vi "ExecuteBuildSpec.vi"(8 "error in (no error)":errorcluster, 10 "Spec Info":T1, 11 "ExecuteAllBuildSpecsWithVersion in":refnum<class "ExecuteAllBuildSpecsWithVersion.lvclass">) -> (0 "error out":errorcluster, 1 "Operation Output/Error Out":string, 2 "CLI Process Return Code":i32, 3 "ExecuteAllBuildSpecsWithVersion out":refnum<class "ExecuteAllBuildSpecsWithVersion.lvclass">)   [LabVIEW 2015, in "ExecuteAllBuildSpecsWithVersion.lvclass"]
doc: "Builds the builds spec in <b>Spec Info</b>."
uses:
  ExecuteAllBuildSpecsWithVersion.lvclass
  ExecuteMultipleBuildSpecs/SpecInformation.ctl
  ExecuteMultipleBuildSpecs/ExecuteMultipleBuildSpecs.lvclass/ExecuteMultipleBuildSpecs.ctl
  <nishared>/LabVIEW CLI/Operations/CoreOperation/CoreOperation.lvclass/CoreOperation.ctl
  ExecuteAllBuildSpecsWithVersion.lvclass/ExecuteAllBuildSpecsWithVersion.ctl
  ExecuteMultipleBuildSpecs/Read Project Path.vi
  <vilib>/AppBuilder/AB_API_Simple/Build (path).vi
  <vilib>/AppBuilder/AB_API_Simple/Set Build Specification Version (path).vi
  <nishared>/LabVIEW CLI/Operations/Utilities/Logger/Logger.lvclass
  <nishared>/LabVIEW CLI/Operations/CoreOperation/CoreOperation.lvclass
  <vilib>/AppBuilder/AB_API_Simple/NI_App_Builder_API.lvlib
  ExecuteMultipleBuildSpecs/ExecuteMultipleBuildSpecs.lvclass
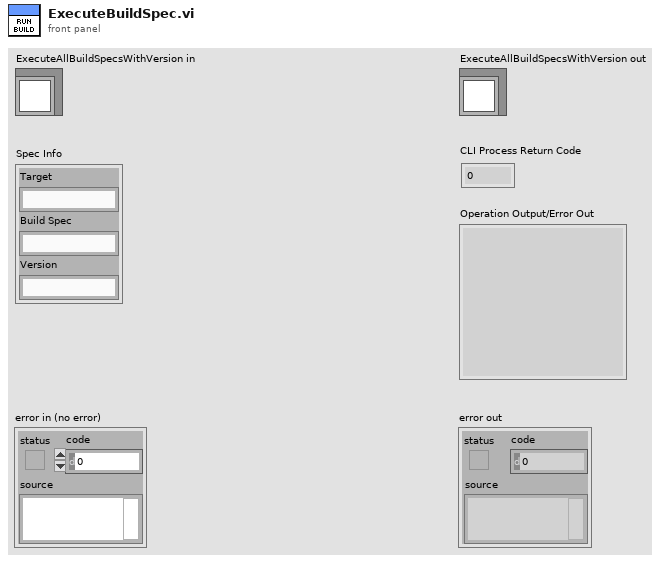
[diagram p1: front panel]
types:
  T1 = typedef "ExecuteMultipleBuildSpecs.lvclass/SpecInformation.ctl" = cluster{"Target":string, "Build Spec":string, "Version":string}
  T2 = typedef "NI_App_Builder_API.lvlib/Build Specification Version.ctl" = cluster{"Major":u16, "Minor":u16, "Fix":u16, "Build":u16}
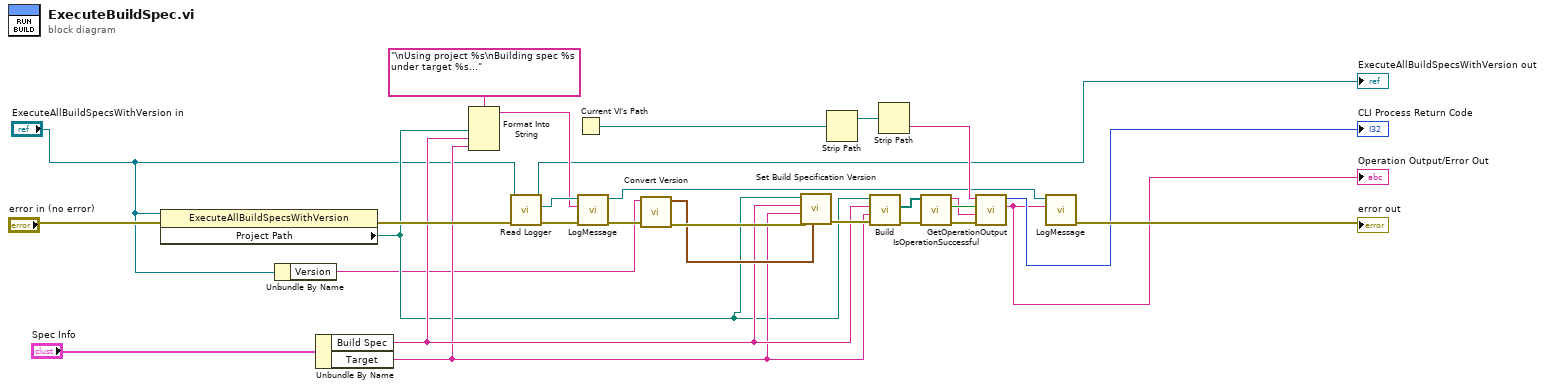
[diagram p0: block diagram]
diagram:
  n1 = property class="ExecuteAllBuildSpecsWithVersion"(reference="ExecuteAllBuildSpecsWithVersion in", error in="error in (no error)") -> (error out=w10:errorcluster, "Project Path"=w3:path)  [unwired: 1 out]
  n2 = Unbundle By Name("ExecuteAllBuildSpecsWithVersion in") -> ("Version"=w1:string)
  n3 = Unbundle By Name("Spec Info") -> ("Build Spec"=w5:string, "Target"=w4:string)
  n4 = Format Into String(format string="\nUsing project %s\nBuilding spec %s under target %s...", w3, w5, w4) -> (resulting string=w26:string)  [unwired: 2 in, 1 out]
  n5 = call <nishared>:"Read Logger.vi"("error in (no error)"=w10, "CoreOperation in"="ExecuteAllBuildSpecsWithVersion in") -> ("error out"=w29:errorcluster, "Logger.lvclass"=w28:refnum<class "Logger.lvclass">, "CoreOperation out"=→"ExecuteAllBuildSpecsWithVersion out":refnum<class "ExecuteAllBuildSpecsWithVersion.lvclass">)  [unwired: 7 in]
  n6 = Current VI's Path() -> (path=w22:path)
  n7 = call <nishared>:"LogMessage.vi"("error in (no error)"=w29, "Message"=w26, "Logger in"=w28) -> ("error out"=w7:errorcluster, "Logger out"=w18:refnum<class "Logger.lvclass">)  [unwired: 7 in]
  n8 = call "Convert Version.vi"("error in (no error)"=w7, "Version"=w1) -> ("error out"=w9:errorcluster, "Build Specification Version"=w8:T2)  [unwired: 8 in]
  n9 = call-poly <vilib>:"Set Build Specification Version.vi"("Build Specification Version"=w8, "error in (no error)"=w9, "Name of target (My Computer)"=w4, "Name of build specification"=w5, "Path to project"=w3) -> ("error out"=w6:errorcluster)  [unwired: 6 in]
  n10 = Strip Path(path=w22) -> (stripped path=w23:path)  [unwired: 1 out]
  n11 = call-poly <vilib>:"Build.vi"("error in (no error)"=w6, "Name of target (My Computer)"=w4, "Name of build specification (if empty: build all)"=w5, "Path to project"=w3) -> ("error out"=w25:errorcluster, "Generated files"=w24:path[])  [unwired: 6 in]
  n12 = Strip Path(path=w23) -> (name=w19:string)  [unwired: 1 out]
  n13 = call "IsOperationSuccessful.vi"("error in (no error)"=w25, "Generated files"=w24) -> ("error out"=w17:errorcluster, "Is Successful?"=w21:bool, "Output/Failure message"=w20:string)  [unwired: 7 in]
  n14 = call <nishared>:"GetOperationOutput.vi"("error in (no error)"=w17, "Operation Output/Error In"=w20, "Operation succeeded?"=w21, "Operation Name"=w19) -> ("Operation Output/Error Out"=w11:string, "CLI Process Return Code"=→"CLI Process Return Code":i32)  [unwired: 6 in]
  "Operation Output/Error Out" <- w11
  n15 = call <nishared>:"LogMessage.vi"("Message"=w11, "Logger in"=w18) -> ("error out"=→"error out":errorcluster)  [unwired: 8 in, 1 out]
